vi "Initialize Hokuyo USB.vi"(8 "error in (no error)":errorcluster, 11 "VISA Refnum in":refnum<visa-resource-name>) -> (0 "error out":errorcluster, 3 "VISA Refnum out":refnum<visa-resource-name>)   [LabVIEW 2016]
doc: "Manually initialize the URG-04LX using USB RAW control commands. Here we treat the device as a Communications Device Class and perform the appropriate initialization routine to emulate Serial commands."
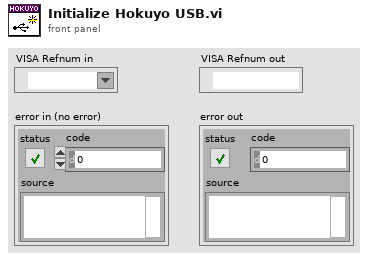
[diagram p1: front panel]
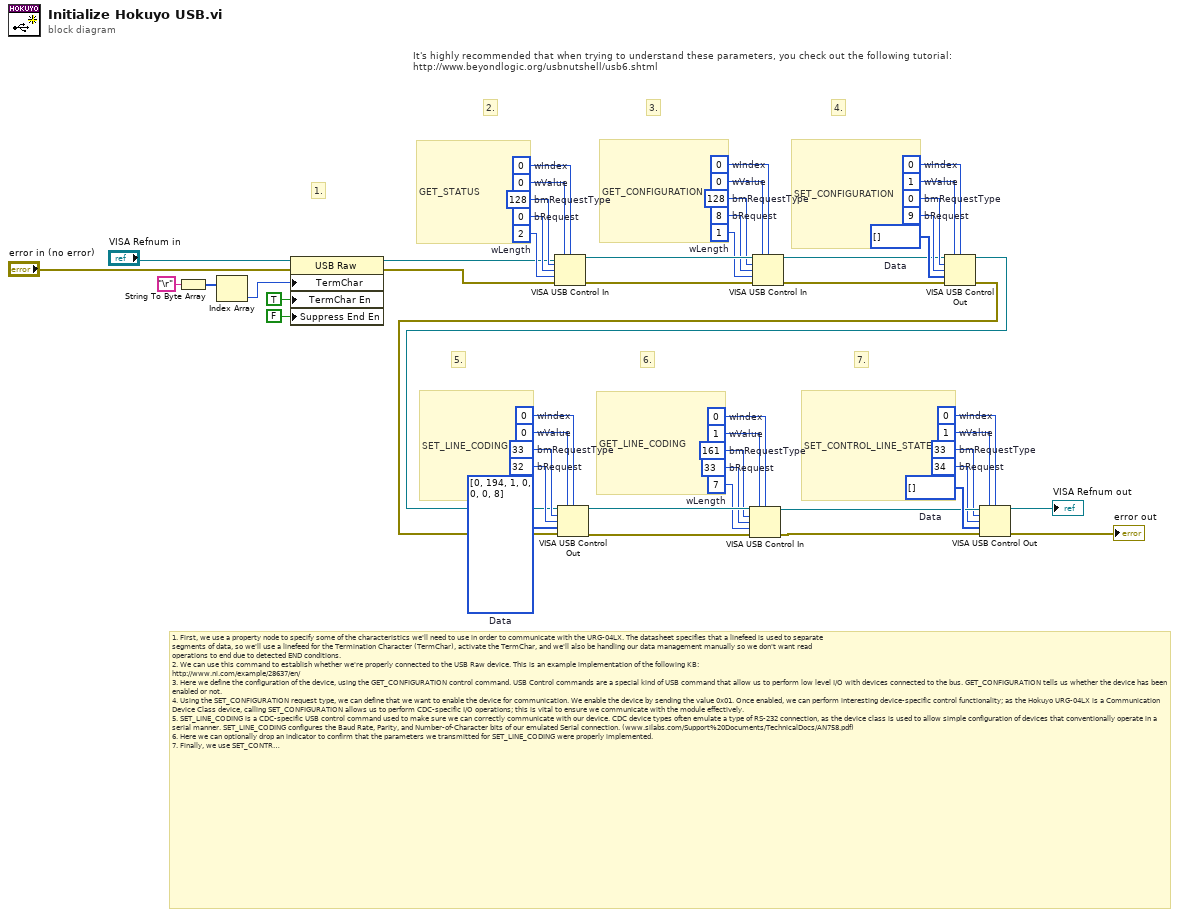
[diagram p0: block diagram]
diagram:
  w49 = u8[] []  # Data
  w43 = u16 0  # wIndex
  w44 = u16 1  # wValue
  w45 = i16 34  # bRequest
  w46 = i16 33  # bmRequestType
  w37 = u16 0  # wIndex
  w36 = u16 1  # wValue
  w40 = u16 7  # wLength
  w39 = i16 33  # bRequest
  w38 = i16 161  # bmRequestType
  w35 = u8[] [0, 194, 1, 0, 0, 0, 8]  # Data
  w34 = u16 0  # wIndex
  w33 = u16 0  # wValue
  w32 = i16 32  # bRequest
  w31 = i16 33  # bmRequestType
  w26 = u8[] []  # Data
  w27 = u16 0  # wIndex
  w28 = u16 1  # wValue
  w30 = i16 9  # bRequest
  w29 = i16 0  # bmRequestType
  w17 = u16 0  # wIndex
  w18 = u16 0  # wValue
  w19 = u16 1  # wLength
  w20 = i16 8  # bRequest
  w21 = i16 128  # bmRequestType
  w16 = u16 0  # wIndex
  w15 = u16 0  # wValue
  w14 = u16 2  # wLength
  w13 = i16 0  # bRequest
  w12 = i16 128  # bmRequestType
  # "It's highly recommended that when trying to understand these parameters, you check out the following tutorial:\nhttp://www.beyondlogic.org/usbnutshell/usb6.shtml"
  # "1. First, we use a property node to specify some of the characteristics we'll need to use in order to communicate with the URG-04LX. The datasheet specifies that a linefeed is used to separate\nsegments of data, so we'll use a linefeed for the Termination Character (TermChar), activate the TermChar, and we'll also be handling our data management manually so we don't want read \noperations to end due to detected END conditions. \n2. We can use this command to establish whether we're properly connected to the USB Raw device. This is an example implementation of the following KB:\nhttp://www.ni.com/example/28637/en/\n3. Here we define the configuration of the device, using the GET_CONFIGURATION control command. USB Control commands are a special kind of USB command that allow us to perform low level I/O with devices connected to the bus. GET_CONFIGURATION tells us whether the device has been enabled or not.\n4. Using the SET_CONFIGURATION request type, we can define that we want to enable the device for communication. We enable the device by sending the value 0x01. Once enabled, we can perform interesting device-specific control functionality; as the Hokuyo URG-04LX is a Communication Device Class device, calling SET_CONFIGURATION allows us to perform CDC-specific I/O operations; this is vital to ensure we communicate with the module effectively.\n5. SET_LINE_CODING is a CDC-specific USB control command used to make sure we can correctly communicate with our device. CDC device types often emulate a type of RS-232 connection, as the device class is used to allow simple configuration of devices that conventionally operate in a serial manner. SET_LINE_CODING configures the Baud Rate, Parity, and Number-of-Character bits of our emulated Serial connection. (www.silabs.com/Support%20Documents/TechnicalDocs/AN758.pdf) \n6. Here we can optionally drop an indicator to confirm that the parameters we transmitted for SET_LINE_CODING were properly implemented. \n7. Finally, we use SET_CONTROL_LINE_STATE; this is used to simply state that the device is now present on the bus, which allows  USB-bulk transfers carrying serial commands to be effectively communicated to the device.\n\nExtra: These parameters for USB configuration cannot be found in the URG-04LX datasheet, or online; they had to be manually captured using USB 'sniffing' software, which allows us to record and analyze USB transactions. The URG-04LX was connected to a test computer, the capture software 'USBlyzer' (http://www.usblyzer.com/) was started, and the software provided with the URG-04LX 'urgBenri' was utilised to start an acquisition that we could monitor. The USB packets transmitted and received during an acquisition were then manually processed in an effort to find which bits we needed to set in order to get LabVIEW to effectively communicate with the device."
  # "7."
  # "6."
  # "5."
  # "4."
  # "3."
  # "2."
  # "1."
  # "SET_CONTROL_LINE_STATE"
  # "GET_LINE_CODING"
  # "SET_LINE_CODING"
  # "SET_CONFIGURATION"
  # "GET_CONFIGURATION"
  # "GET_STATUS"
  n1 = String To Byte Array(string="\r") -> (unsigned byte array=w8:u8[])
  n2 = Index Array(array=w8) -> (element=w7:u8)  [unwired: 1 in]
  n3 = property class="USB Raw"(reference="VISA Refnum in", error in="error in (no error)", "TermChar"=w7, "TermChar En"=TRUE ("Message Based Settings:Termination Character Enable"), "Suppress End En"=FALSE ("Message Based Settings:Suppress End Enable")) -> (reference out=w4:refnum<visa-resource-name>, error out=w3:errorcluster)
  n4 = VISA USB Control In(0:w4, 1:w15, 2:w16, 5:w12, 7:w13, 9:w14, 11:w3) -> (4:w22:refnum<visa-resource-name>, 15:w23:errorcluster)  [unwired: 1 out]
  n5 = VISA USB Control In(0:w22, 1:w18, 2:w17, 5:w21, 7:w20, 9:w19, 11:w23) -> (4:w24:refnum<visa-resource-name>, 15:w25:errorcluster)  [unwired: 1 out]
  n6 = VISA USB Control Out(0:w24, 1:w28, 2:w27, 5:w29, 7:w30, 9:w26, 11:w25) -> (4:w2:refnum<visa-resource-name>, 15:w1:errorcluster)
  n7 = VISA USB Control Out(0:w2, 1:w33, 2:w34, 5:w31, 7:w32, 9:w35, 11:w1) -> (4:w41:refnum<visa-resource-name>, 15:w42:errorcluster)
  n8 = VISA USB Control In(0:w41, 1:w36, 2:w37, 5:w38, 7:w39, 9:w40, 11:w42) -> (4:w47:refnum<visa-resource-name>, 15:w48:errorcluster)  [unwired: 1 out]
  n9 = VISA USB Control Out(0:w47, 1:w44, 2:w43, 5:w46, 7:w45, 9:w49, 11:w48) -> (4:→"VISA Refnum out":refnum<visa-resource-name>, 15:→"error out":errorcluster)
